vi "Get Single ID Only By Filter.vi"(8 "error in (no error)":errorcluster, 10 "Table ID":u32=508, 11 "Filter":T1={"Field Name"="Full PN", "Filter Type"="contains", "Filter Value"="80-00000"}) -> (0 "error out":errorcluster, 3 "ID":i32=235)   [LabVIEW 2018]
uses:
  TypeDef/FIlter.ctl
  <vilib>/Utility/error.llb/Error Cluster From Error Code.vi
  <vilib>/ErrorRing/Error Ring.xnode
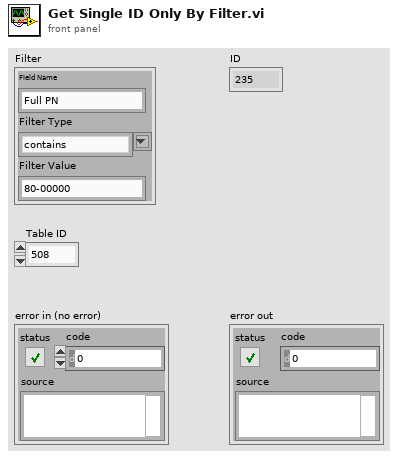
[diagram p1: front panel]
types:
  T1 = typedef "FIlter.ctl" = cluster{"Field Name":string, "Filter Type":string, "Filter Value":string}
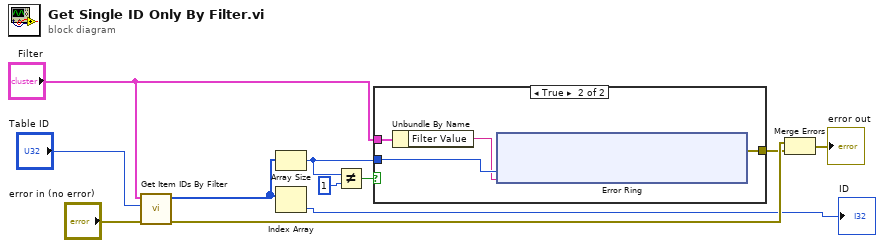
[diagram p0: block diagram]
diagram:
  n1 = call "Get Item IDs By Filter.vi"("error in (no error)"="error in (no error)", "Table ID"="Table ID", "Filter"="Filter") -> ("error out"=w10:errorcluster, "Item IDs"=w1:i32[])  [unwired: 7 in]
  n2 = Array Size(array=w1) -> (size(s)=w3:i32)
  n3 = Index Array(array=w1) -> (element=→"ID":i32)  [unwired: 1 in]
  n4 = Not Equal?(x=w3, y=1) -> (x != y?=w7:bool)
  n5 = case shown="True" w7 {
    tunnel: [_ w15] -> w4
    tunnel: w3 -> [_ w14]
    tunnel: "Filter" -> [_ w13]
    frame False {
    }
    frame True {
      n6 = Unbundle By Name(w13) -> ("Filter Value"=w12:string)
      n7 = xnode "Error Ring"("parameter 0"=w14, "parameter 1"=w12) -> ("error out"=w15:errorcluster)
    }
  }
  n8 = Merge Errors(w10, w4) -> (→"error out":errorcluster)
